vi "XIPIN_Simulation_Clock_Generator_1_0.vi"   [LabVIEW 2017]
doc: "Simulation only CLOCK Generator. The core generates Differential or Single Ended clock signal.\n------------------------------------\n<b>Need License</b> : No"
uses:
  <vilib>/rvi/XilinxIP/XIPIN_XNode/niFpgaXIPIN.xnode
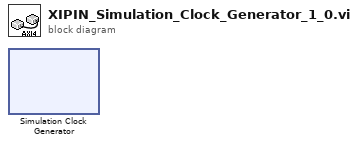
[diagram p0: block diagram]
diagram:
  n1 = xnode ("Simulation Clock Generator")() -> ()
